vi "Get FIFOs Indexes.vi"(8 "error in (no error)":errorcluster, 10 "Channels Refs":T3[](array[typedef]) {"Array of Refs" format="%.0x"}, 11 "Device Ref in":T4=18446744073709551615 format="%.0x") -> (0 "error out":errorcluster, 2 "Array":T1[](array[typedef]))   [LabVIEW 2014, in "Modbus System Explorer.lvlib"]
uses:
  Modbus System Explorer.lvlib
  <vilib>/NI Veristand/Custom Device API/Custom Device Item Ref.ctl
  Shared/Channels Ref.ctl
  Shared/FIFO Indexes.ctl
  <vilib>/NI Veristand/Custom Device API/Custom Device Channel Type.ctl
  <vilib>/NI Veristand/Custom Device Tools/Custom Device Utility Library/Custom Device Utility Library.lvlib
  Shared/Modbus Shared.lvlib
  <vilib>/NI Veristand/Custom Device API/Custom Device API.lvlib
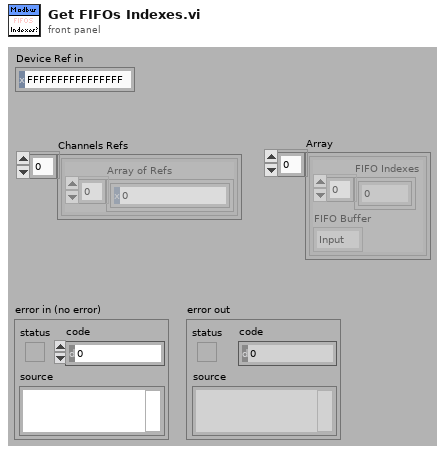
[diagram p1: front panel]
types:
  T1 = typedef "Modbus Shared.lvlib/FIFO Indexes.ctl" = cluster{"FIFO Indexes":i32[], "FIFO Buffer":T2}
  T2 = typedef "Custom Device API.lvlib/Custom Device Channel Type.ctl" = enum16{"Input", "Output"}
  T3 = typedef "Modbus Shared.lvlib/Channels Ref.ctl" = cluster{"Array of Refs":T4[]}
  T4 = typedef "Custom Device API.lvlib/Custom Device Item Ref.ctl" = u64
  T5 = cluster{"status":bool, "code":i32, "source 2":string}
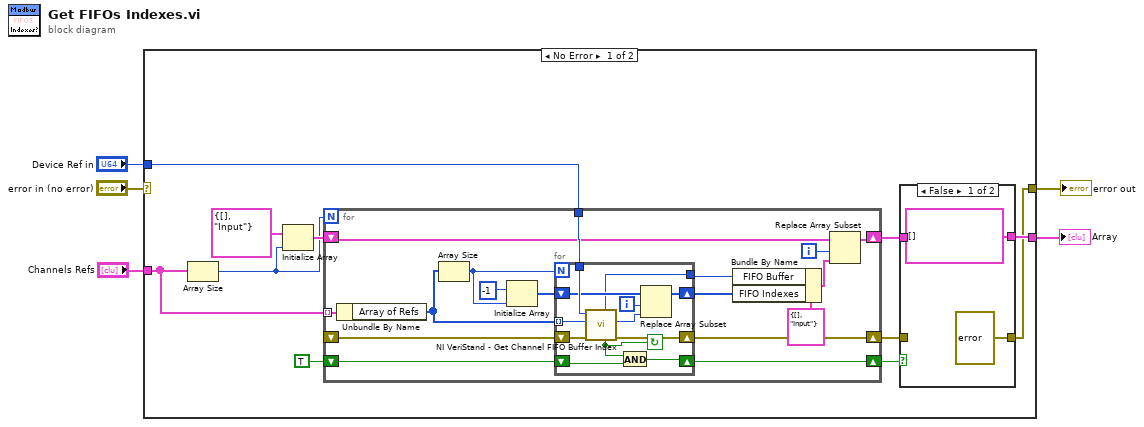
[diagram p0: block diagram]
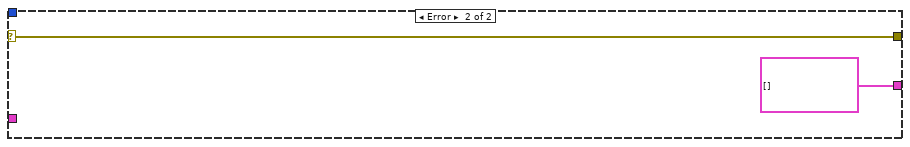
[diagram p3: hidden frame]
diagram:
  n1 = case shown="No Error" "error in (no error)" {
    selector: "error in (no error)" -> [_ w51]
    tunnel: [w6 w51] -> w5
    tunnel: "Device Ref in" -> [w8 _]
    tunnel: "Channels Refs" -> [w16 _]
    tunnel: [w7 T1[] []] -> w1
    frame No Error {
      n2 = Array Size(array=w16) -> (size(s)=w13:i32)
      n3 = Initialize Array(T1 {"FIFO Indexes"=[], "FIFO Buffer"=enum."Input"} ("Cluster"), w13) -> (w14:T1[])
      n4 = for {
        N: w13 -> [_]
        tunnel: w8 -> [w37]
        shift-right: [w35] -> w9
        shift-left: w14 -> [w36]
        tunnel: w16 -> [w31] mode=indexing
        shift-right: [w24] -> w10
        shift-left: _ -> [w29]
        shift-right: [w21] -> w11
        shift-left: TRUE -> [w22]
        i -> [w34]
        n5 = Unbundle By Name(w31) -> ("Array of Refs"=w30:T4[])
        n6 = Array Size(array=w30) -> (size(s)=w27:i32)
        n7 = Initialize Array(-1, w27) -> (w26:i32[])
        n8 = for {
          N: w27 -> [_]
          tunnel: w37 -> [w49]
          tunnel: w30 -> [w39] mode=indexing
          shift-right: [w46] -> w25
          shift-left: w26 -> [w47]
          shift-right: [w44] -> w24
          shift-left: w29 -> [w48]
          tunnel: [w43] -> w23
          shift-right: [w40] -> w21
          shift-left: w22 -> [w41]
          i -> [w45]
          stop <- w42 continue-if-true
          n9 = call <vilib>:"NI VeriStand - Get Channel FIFO Buffer Index.vi"("error in"=w48, "Channel Ref"=w39, "Device Ref in"=w49) -> ("error out"=w44:errorcluster, "Channel FIFO Buffer Index"=w38:i32, "Found"=w42:bool, "FIFO Buffer"=w43:T2)  [unwired: 4 in, 1 out]
          n10 = And(x=w42, y=w41) -> (x .and. y?=w40:bool)
          n11 = Replace Array Subset(array=w47, new element=w38, index=w45) -> (w46:i32[])
        }
        n12 = Bundle By Name(cluster=T1 {"FIFO Indexes"=[], "FIFO Buffer"=enum."Input"} ("Cluster"), "FIFO Buffer"=w23, "FIFO Indexes"=w25) -> (w33:T1)
        n13 = Replace Array Subset(array=w36, new element=w33, index=w34) -> (w35:T1[])
      }
      n14 = case shown="False" w11 {
        tunnel: w10 -> [_ w20]
        tunnel: [T5 {"status"=TRUE, "code"=5025, "source 2"="Action VI On Compile: couldn't find all FIFO Indexes."} ("error IO") w20] -> w6
        tunnel: w9 -> [_ w19]
        tunnel: [T1[] [] w19] -> w7
        frame False {
        }
        frame True {
        }
      }
    }
    frame Error {
    }
  }
  "error out" <- w5
  "Array" <- w1
